vi "cvt_Enum_MemBlock.vi"(8 "Value":i32, 9 "Index":i32, 10 "Default Data":i32[](array[numeric]), 11 "Method":T1=enum."read") -> (0 "Value":i32, 2 "AllData":i32[](array[numeric]))   [LabVIEW 2020, in "Current Value Table(Rebuild).lvlib"]
uses:
  Current Value Table(Rebuild).lvlib
  TypeDefs/cvt_MemBlock Methods.ctl
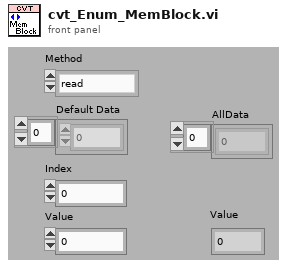
[diagram p1: front panel]
types:
  T1 = typedef "Current Value Table(Rebuild).lvlib/cvt_MemBlock Methods.ctl" = enum16{"init", "read", "readall", "write"}
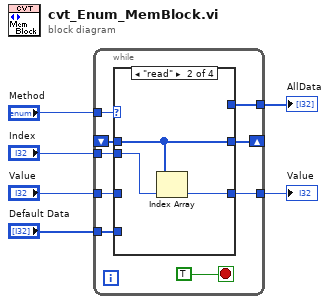
[diagram p0: block diagram]
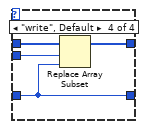
[diagram p4: hidden frame]
diagram:
  n1 = while {
    shift-right: [w13] -> _
    shift-left: _ -> [w12]
    tunnel: "Method" -> [w14]
    tunnel: "Value" -> [w11]
    tunnel: [w10] -> w4
    tunnel: "Index" -> [w9]
    tunnel: [w8] -> w2
    tunnel: "Default Data" -> [w7]
    stop <- TRUE stop-if-true
    n2 = case shown="\"read\"" w14 {
      tunnel: [w16 w19 w20 w24] -> w13
      tunnel: w12 -> [_ w19 w20 w22]
      tunnel: w11 -> [_ _ _ w23]
      tunnel: [_ w18 _ w23] -> w10
      tunnel: w9 -> [_ w17 _ w21]
      tunnel: [_ _ w20 _] -> w8
      tunnel: w7 -> [w16 _ _ _]
      frame "init" {
      }
      frame "read" {
        n3 = Index Array(array=w19, index=w17) -> (element=w18:i32)
      }
      frame "readall" {
      }
      frame "write", Default {
        n4 = Replace Array Subset(array=w22, new element=w23, index=w21) -> (w24:i32[])
      }
    }
  }
  "Value" <- w4
  "AllData" <- w2
